vi "Format_specifier.vi"() -> ()   [LabVIEW 2019]
panel:
  in  "Event":string="National Technology Day"
  in  "Time":i32=100
  in  "Temperature":dbl=37.52
  in  "Date":i32=11
  out "Output":string
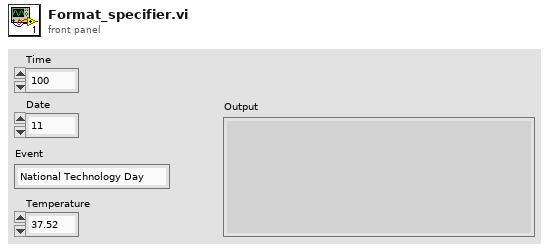
[diagram p1: front panel]
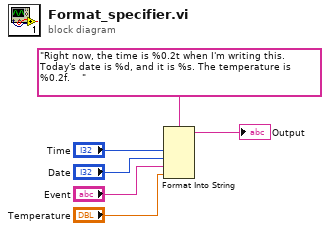
[diagram p0: block diagram]
diagram:
  n1 = Format Into String(format string="Right now, the time is %0.2t when I'm writing this. Today's date is %d, and it is %s. The temperature is %0.2f.    ", "Time", "Date", "Event", "Temperature") -> (resulting string=→"Output":string)  [unwired: 2 in, 1 out]
